vi "Create.vi"(8 "error in (no error)":errorcluster, 11 "Mermaid":string) -> (0 "error out":errorcluster, 3 "ParseMermaid out":refnum<class "ParseMermaid.lvclass">)   [LabVIEW 2020, in "Mermaid.lvlib" / "ParseMermaid.lvclass"]
uses:
  ParseMermaid.lvclass
  ParseMermaid.lvclass/ParseMermaid.ctl
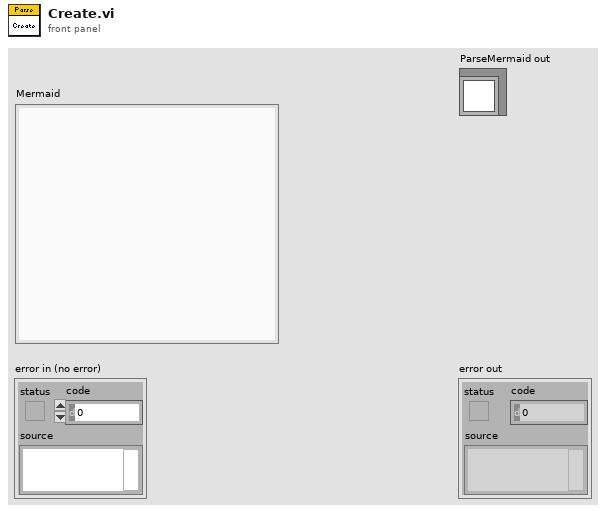
[diagram p1: front panel]
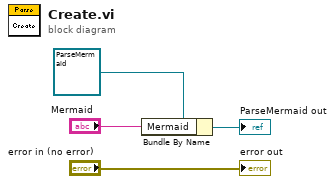
[diagram p0: block diagram]
diagram:
  n1 = Bundle By Name(cluster=refnum<class "ParseMermaid.lvclass"> refnum ("ParseMermaid out"), "Mermaid"="Mermaid") -> (→"ParseMermaid out":refnum<class "ParseMermaid.lvclass">)
  "error out" <- "error in (no error)"
